vi "Update Driver Settings.vi"(8 "error in (no error)":errorcluster, 9 "Command Settings":refnum<class "CommandSetting.lvclass">[](array[class]), 10 "Command Id":string, 11 "Driver in":refnum<class "Driver.lvclass">) -> (0 "error out":errorcluster, 1 "Settings Updated":u32, 2 "Settings Added":u32, 3 "Driver out":refnum<class "Driver.lvclass">)   [LabVIEW 2023, in "HAF.lvlib" / "Driver.lvclass"]
doc: "Updates the Driver Settings collection from the given Command Settings. These are mapped first. Reports on the number added and the number updated."
uses:
  Driver.lvclass
  Driver.lvclass/Driver.ctl
  DriverSetting/DriverSetting.lvclass
  CommandSetting/CommandSetting.lvclass
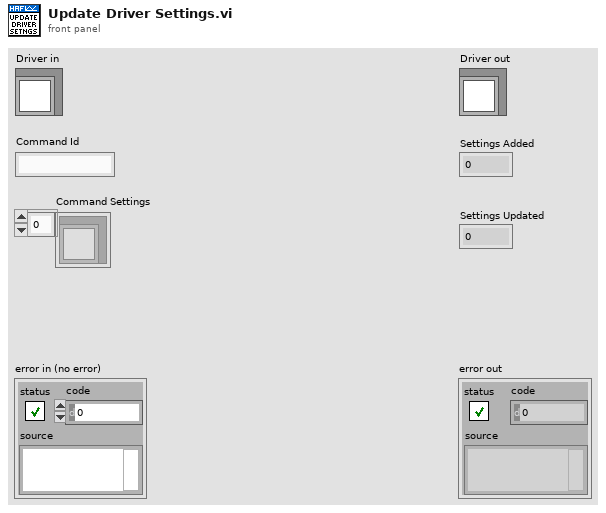
[diagram p1: front panel]
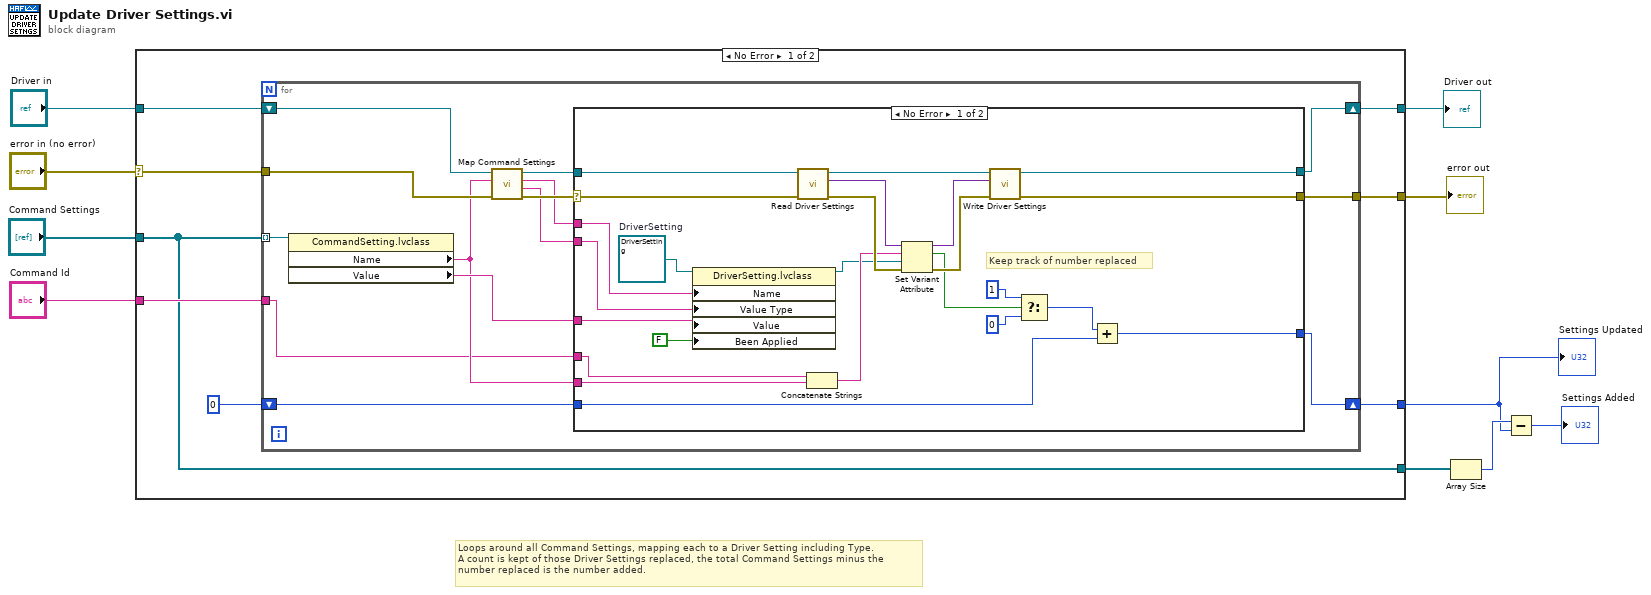
[diagram p0: block diagram]
diagram:
  # "Loops around all Command Settings, mapping each to a Driver Setting including Type.\nA count is kept of those Driver Settings replaced, the total Command Settings minus the\nnumber replaced is the number added."
  n1 = case shown="No Error" "error in (no error)" {
    selector: "error in (no error)" -> [w17 w60]
    tunnel: [w14 w60] -> w5
    tunnel: [w15 w59] -> w6
    tunnel: "Driver in" -> [w18 w59]
    tunnel: "Command Settings" -> [w12 _]
    tunnel: "Command Id" -> [w13 _]
    tunnel: [w12 _] -> w4
    tunnel: [w11 _] -> w1
    frame No Error {
      n2 = for {
        shift-right: [w19] -> w15
        shift-left: w18 -> [w31]
        tunnel: w17 -> [w30]
        tunnel: w12 -> [w32] mode=indexing
        shift-right: [w21] -> w11
        shift-left: u32 0 ("Number Replaced") -> [w23]
        tunnel: w13 -> [w22]
        tunnel: [w20] -> w14
        n3 = property class="CommandSetting.lvclass"(reference=w32) -> ("Name"=w24:string, "Value"=w25:string)  [unwired: 1 in, 2 out]
        n4 = call-dynamic "Map Command Settings.vi"("error in (no error)"=w30, "Command Setting Name"=w24, "Driver in"=w31) -> ("error out"=w28:errorcluster, "Setting Data Type"=w26:string, "Mapped Driver Name"=w27:string, "Driver out"=w29:refnum<class "Driver.lvclass">)  [unwired: 5 in]
        n5 = case shown="No Error" w28 {
          selector: w28 -> [w48 w57]
          tunnel: w29 -> [w49 w58]
          tunnel: [w40 w58] -> w19
          tunnel: [w39 w57] -> w20
          tunnel: w27 -> [w55 _]
          tunnel: w26 -> [w54 _]
          tunnel: w25 -> [w53 _]
          tunnel: w24 -> [w50 _]
          tunnel: w23 -> [w34 _]
          tunnel: w22 -> [w51 _]
          tunnel: [w33 _] -> w21
          frame No Error {
            w56 = refnum<class "DriverSetting.lvclass"> refnum  # DriverSetting
            # "Keep track of number replaced"
            n6 = property class="DriverSetting.lvclass"(reference=w56, "Name"=w55, "Value Type"=w54, "Value"=w53, "Been Applied"=FALSE) -> (reference out=w44:refnum<class "DriverSetting.lvclass">)  [unwired: 1 in, 1 out]
            n7 = call-dynamic "Read Driver Settings.vi"("error in (no error)"=w48, "Driver in"=w49) -> ("error out"=w46:errorcluster, "Driver Settings"=w47:variant, "Driver out"=w43:refnum<class "Driver.lvclass">)  [unwired: 7 in]
            n8 = Concatenate Strings(w51, w50) -> (w45:string)
            n9 = Set Variant Attribute(Variant=w47, name=w45, value=w44, error in=w46) -> (Variant out=w41:variant, replaced=w38:bool, error out=w42:errorcluster)
            n10 = call-dynamic "Write Driver Settings.vi"("error in (no error)"=w42, "Driver Settings"=w41, "Driver in"=w43) -> ("error out"=w39:errorcluster, "Driver out"=w40:refnum<class "Driver.lvclass">)  [unwired: 7 in]
            n11 = Select(t=u32 1, s=w38, f=u32 0) -> (s? t:f=w35:u32)
            n12 = Add(x=w35, y=w34) -> (x+y=w33:u32)
          }
          frame Error {
          }
        }
      }
    }
    frame Error {
    }
  }
  "error out" <- w5
  "Driver out" <- w6
  "Settings Updated" <- w1
  n13 = Array Size(array=w4) -> (size(s)=w3:i32)
  n14 = Subtract(x=w3, y=w1) -> (x-y=→"Settings Added":u32)
